vi "ThrowError.vi"(8 "error in (no error)":errorcluster, 10 "current error in":errorcluster, 11 "Boolean":bool) -> (0 "error out":errorcluster)   [LabVIEW 2014]
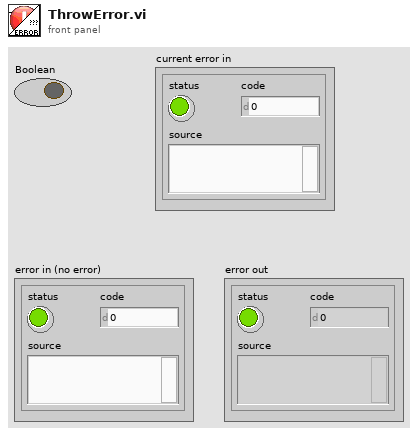
[diagram p1: front panel]
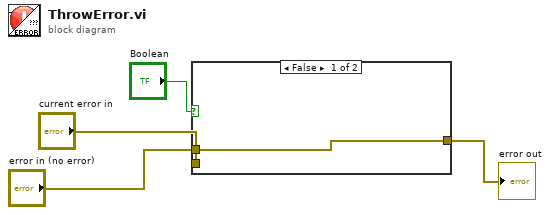
[diagram p0: block diagram]
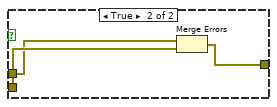
[diagram p2: hidden frame]
diagram:
  n1 = case shown="False" "Boolean" {
    tunnel: "error in (no error)" -> [w5 w7]
    tunnel: [w5 w6] -> w4
    tunnel: "current error in" -> [_ w8]
    frame False {
    }
    frame True {
      n2 = Merge Errors(w7, w8) -> (w6:errorcluster)
    }
  }
  "error out" <- w4
